vi "Get Sampling.vi"(8 "error in (no error)":errorcluster, 11 "DAQmx in":refnum<class "DAQmx.lvclass">) -> (0 "error out":errorcluster, 2 "Sampling info":T1 {"Fs" format="%#_13g"}, 3 "DAQmx out":refnum<class "DAQmx.lvclass">)   [LabVIEW 2019, in "DAQmx.lvclass"]
uses:
  DAQmx.lvclass
  typedefs/DAQ.Config.Timing.Sampling--Cluster.ctl
  DAQmx.lvclass/DAQmx.ctl
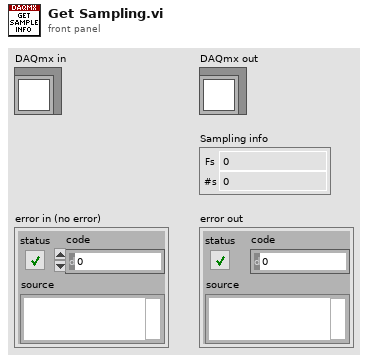
[diagram p1: front panel]
types:
  T1 = typedef "DAQmx.lvclass/DAQ.Config.Timing.Sampling--Cluster.ctl" = cluster{"Fs":dbl, "#s":i32}
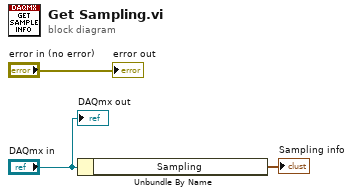
[diagram p0: block diagram]
diagram:
  n1 = Unbundle By Name("DAQmx in") -> ("Sampling"=→"Sampling info":T1)
  "error out" <- "error in (no error)"
  "DAQmx out" <- "DAQmx in"
